vi "Misc Variable.vi"() -> ()   [LabVIEW 2010]
panel:
  in  "Misc Variable":dbl[](array[numeric])
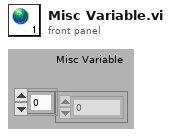
[diagram p1: front panel]
diagram:
